vi "Close Device Core.vi"(8 "error in (no error)":errorcluster, 11 "IVI_DMM_Delayed in":refnum<class "IVI_DMM_Delayed.lvclass">) -> (0 "error out":errorcluster, 3 "IVI_DMM_Delayed out":refnum<class "IVI_DMM_Delayed.lvclass">)   [LabVIEW 2015, in "IVI_DMM.lvlib" / "IVI_DMM_Delayed.lvclass"]
doc: "Close device driver connection."
uses:
  IVI_DMM_Delayed.lvclass
  IVI_DMM_Delayed.lvclass/IVI_DMM_Delayed.ctl
  IVI_DMM/IVI_DMM.lvclass
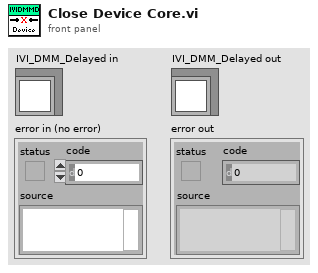
[diagram p1: front panel]
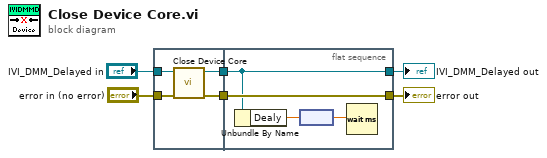
[diagram p0: block diagram]
diagram:
  n1 = flat-sequence {
    tunnel: "error in (no error)" -> [w8]
    tunnel: "IVI_DMM_Delayed in" -> [w7]
    tunnel: [w10] -> w2
    tunnel: [w9] -> w1
    tunnel: [w13] -> w5
    tunnel: [w14] -> w6
    tunnel: w2 -> [w14]
    tunnel: w1 -> [w13]
    frame #0 {
      n2 = call-parent "Close Device Core.vi"("error in (no error)"=w8, "IVI_DMM in"=w7) -> ("error out"=w10:errorcluster, "IVI_DMM out"=w9:refnum<class "IVI_DMM_Delayed.lvclass">)  [unwired: 8 in]
    }
    frame #1 {
      n3 = Unbundle By Name(w13) -> ("Dealy"=w12:dbl[unit])
      n4 = node(w12) -> (w11:dbl)
      n5 = Wait (ms)(milliseconds to wait=w11) -> ()  [unwired: 1 out]
    }
  }
  "error out" <- w6
  "IVI_DMM_Delayed out" <- w5
